vi "RealTime_Main.vi"() -> ()   [LabVIEW 2019]
uses:
  <vilib>/FPGAPlugInAG/sbRIO-9628/niLvFpga_Open_sbRIO-9628.vi
  <vilib>/rvi/interface/common/dynamic/niFpgaDynamicAddResources.vi
  <vilib>/Utility/error.llb/Error Cluster From Error Code.vi
  <vilib>/rvi/errors/niLvFpgaAdjustHostInterfaceError.vi
  <vilib>/FPGAPlugInAG/Dynamic/niLvFpga_Close_Dynamic.vi
  <vilib>/rvi/interface/nirviOpenFPGA/nirviOpenFPGA.xnode
  FPGA/build/aerialladdertruc_FPGATarget_FPGAMain_I0aLQvUnu8Y.lvbitx
  FPGA/FPGA_Main.vi
  <vilib>/rvi/interface/nirviReadWriteControl/nirviReadWriteControl.xnode
  <vilib>/rvi/interface/nirviCloseFPGA/nirviCloseFPGA.xnode
  NiFpgaLv.dll
  <vilib>/rvi/interface/Simulation/niFpgaSimulationCallBeginRW.vi
panel:
  out "XY Graph 2":cluster{dbl[], dbl[]}[](graph)
  in  "Stop":bool
  out "ZMP_X-Axis_Position(mm)":dbl format="%.1f"
  out "ZMP_Y-Axis_Position(mm)":dbl format="%.1f"
  out "HeartBeatSignal":bool
  in  "Ladeer_Mass(Kg)":dbl=3726.0 format="%.1f"
  in  "Ladeer_Mass_Point(mm)":dbl=10500.0 format="%.1f"
  in  "Load(Kg)":dbl=653.7 format="%.1f"
  in  "Outrigger_Front_Position(mm)":dbl=3264.0 format="%.1f"
  in  "Outrigger_Rear_Position(mm)":dbl=-30.0 format="%.1f"
  in  "Outrigger_RR_Length(mm)":dbl=1990.0 format="%.1f"
  in  "Outrigger_RL_Length(mm)":dbl=-1990.0 format="%.1f"
  in  "Outrigger_FR_Length(mm)":dbl=2050.0 format="%.1f"
  in  "Outrigger_FL_Length(mm)":dbl=-2050.0 format="%.1f"
  in  "Vehicle_Mass(Kg)":dbl=13427.0 format="%.1f"
  in  "Boom_Rising_Angle(Degree)":dbl
  in  "Boom_Rotation_Angle(Degree)":dbl format="%.1f"
  # "Aerial Ladder Truck Monitoring Program"
  # "Vehicle Parameter"
  # "Sensor Parameter"
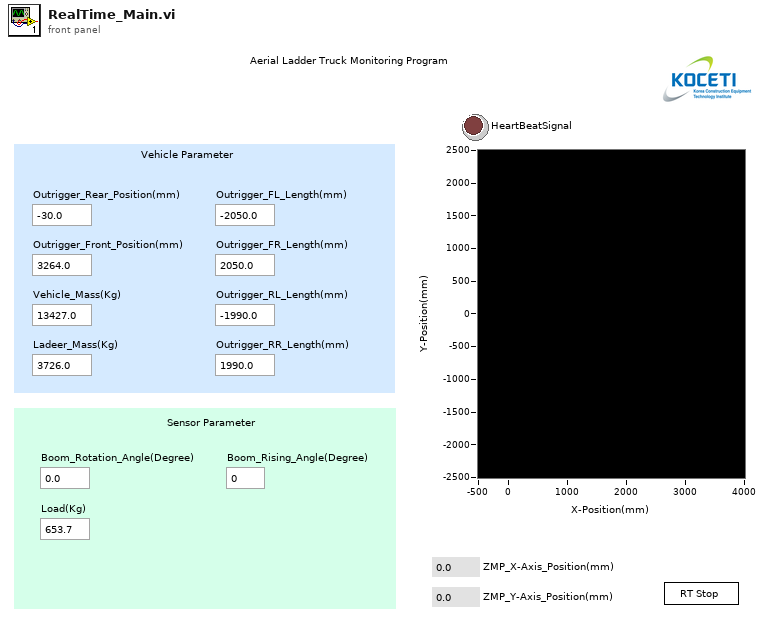
[diagram p1: front panel]
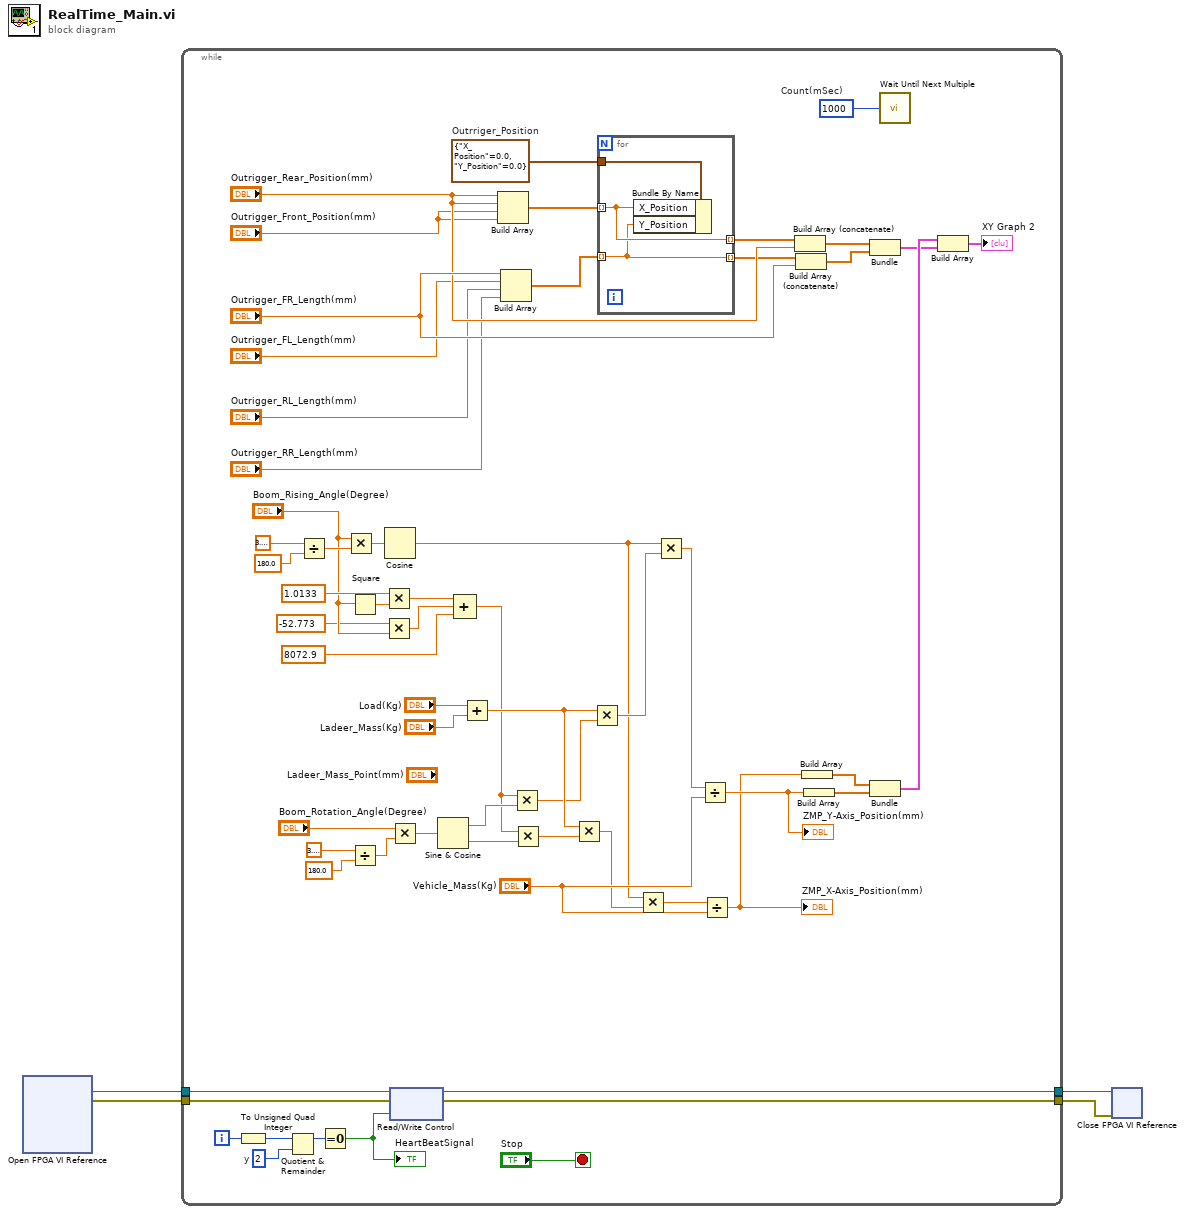
[diagram p0: block diagram]
diagram:
  n1 = xnode "Open FPGA VI Reference"() -> ("FPGA VI Reference Out"=w4:refnum<k20>, "error out"=w3:errorcluster)  [unwired: 2 in]
  n2 = while {
    tunnel: w4 -> [w49]
    tunnel: w3 -> [w47]
    tunnel: [w44] -> w2
    tunnel: [w43] -> w1
    i -> [w38]
    stop <- "Stop" stop-if-true
    w24 = cluster{"X_Position":dbl, "Y_Position":dbl} {"X_Position"=0.0, "Y_Position"=0.0}  # Outrriger_Position
    w46 = u64 2  # y
    w48 = u32 1000  # Count(mSec)
    n3 = To Unsigned Quad Integer(1:w38) -> (0:w37:u64)
    n4 = Quotient & Remainder(x=w37, y=w46) -> (x-y*floor(x/y)=w45:u64)  [unwired: 1 out]
    n5 = Divide(x=3.141592653589793, y=180.0) -> (x/y=w20:dbl)
    n6 = Equal To 0?(x=w45) -> (x = 0?=w42:bool)
    "HeartBeatSignal" <- w42
    n7 = Multiply(x="Boom_Rising_Angle(Degree)", y=w20) -> (x*y=w19:dbl)
    n8 = Square(x="Boom_Rising_Angle(Degree)") -> (x^2=w12:dbl)
    n9 = Divide(x=3.141592653589793, y=180.0) -> (x/y=w62:dbl)
    n10 = Multiply(x=1.0133, y=w12) -> (x*y=w8:dbl)
    n11 = Multiply(x=-52.773, y="Boom_Rising_Angle(Degree)") -> (x*y=w7:dbl)
    n12 = Cosine(x=w19) -> (cos(x)=w16:dbl)
    n13 = Multiply(x="Boom_Rotation_Angle(Degree)", y=w62) -> (x*y=w63:dbl)
    n14 = xnode "Read/Write Control"("FPGA VI Reference In"=w49, "error in"=w47, "Signal"=w42) -> ("FPGA VI Reference Out"=w44:refnum<k20>, "error out"=w43:errorcluster)
    n15 = Sine & Cosine(0:w63) -> (1:w55:dbl, 2:w58:dbl)
    n16 = Compound Arithmetic op=ADD(w8, w7, 8072.9) -> (w5:dbl)
    n17 = Add(x="Load(Kg)", y="Ladeer_Mass(Kg)") -> (x+y=w56:dbl)
    n18 = Build Array("Outrigger_Rear_Position(mm)", "Outrigger_Rear_Position(mm)", "Outrigger_Front_Position(mm)", "Outrigger_Front_Position(mm)") -> (w25:dbl[])
    n19 = Build Array("Outrigger_FR_Length(mm)", "Outrigger_FL_Length(mm)", "Outrigger_RL_Length(mm)", "Outrigger_RR_Length(mm)") -> (w26:dbl[])
    n20 = Multiply(x=w5, y=w55) -> (x*y=w54:dbl)
    n21 = Multiply(x=w5, y=w58) -> (x*y=w57:dbl)
    n22 = Multiply(x=w56, y=w57) -> (x*y=w15:dbl)
    n23 = Multiply(x=w56, y=w54) -> (x*y=w18:dbl)
    n24 = for {
      tunnel: w25 -> [w67] mode=indexing
      tunnel: w24 -> [w68]
      tunnel: w26 -> [w66] mode=indexing
      tunnel: [w67] -> w31 mode=indexing
      tunnel: [w66] -> w32 mode=indexing
      n25 = Bundle By Name(cluster=w68, "X_Position"=w67, "Y_Position"=w66) -> ()  [unwired: 1 out]
    }
    n26 = Multiply(x=w16, y=w15) -> (x*y=w14:dbl)
    n27 = Multiply(x=w16, y=w18) -> (x*y=w17:dbl)
    n28 = Divide(x=w17, y="Vehicle_Mass(Kg)") -> (x/y=w41:dbl)
    "ZMP_Y-Axis_Position(mm)" <- w41
    n29 = Divide(x=w14, y="Vehicle_Mass(Kg)") -> (x/y=w40:dbl)
    "ZMP_X-Axis_Position(mm)" <- w40
    n30 = Build Array (concatenate)(w31, "Outrigger_Rear_Position(mm)") -> (w35:dbl[])
    n31 = Build Array (concatenate)(w32, "Outrigger_FR_Length(mm)") -> (w36:dbl[])
    n32 = Build Array(w40) -> (w51:dbl[])
    n33 = Build Array(w41) -> (w52:dbl[])
    n34 = Bundle(w35, w36) -> (w23:cluster{dbl[], dbl[]})  [unwired: 1 in]
    n35 = Bundle(w51, w52) -> (w50:cluster{dbl[], dbl[]})  [unwired: 1 in]
    n36 = call "Wait Until Next Multiple"("Count(mSec)"=w48) -> ()  [unwired: 1 out]
    n37 = Build Array(w50, w23) -> (→"XY Graph 2":cluster{dbl[], dbl[]}[])
  }
  n38 = xnode "Close FPGA VI Reference"("FPGA VI Reference In"=w2, "error in"=w1) -> ()  [unwired: 1 out]
